vi "MyMethod2.vi"(0 "reference in":refnum<class "AnotherClass.lvclass">, 5 "error in (no error)":errorcluster) -> (14 "reference out":refnum<class "AnotherClass.lvclass">, 19 "error out":errorcluster)   [LabVIEW 2017, in "AnotherClass.lvclass"]
uses:
  AnotherClass.lvclass
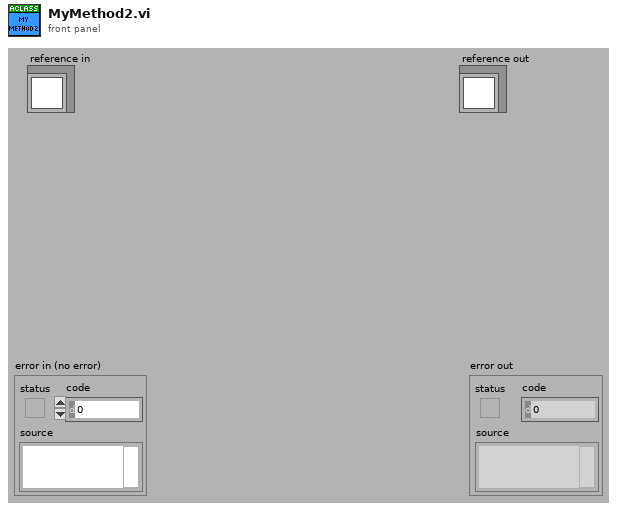
[diagram p1: front panel]
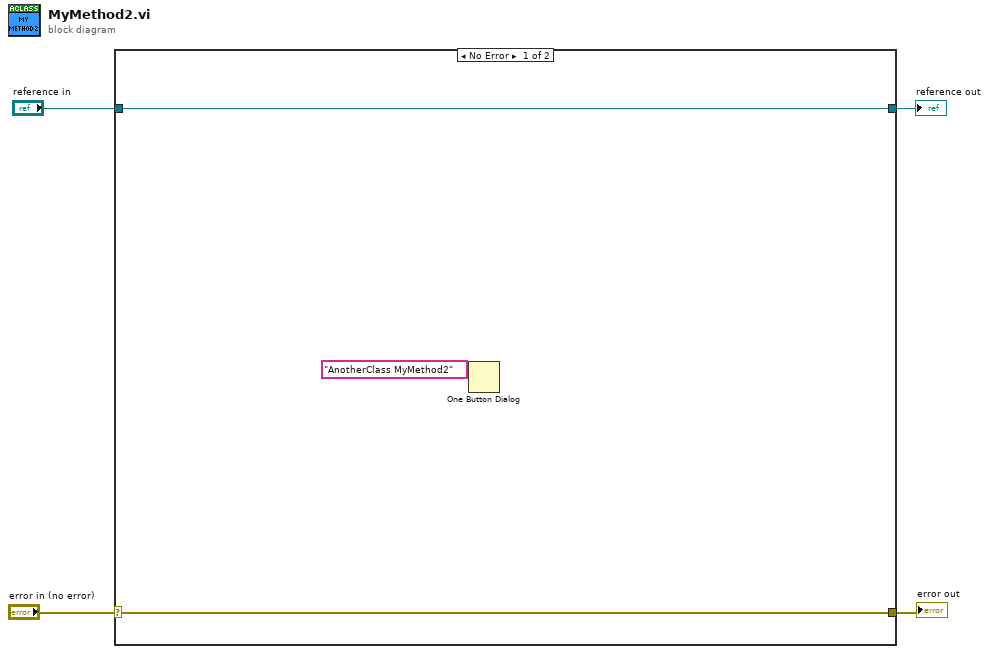
[diagram p0: block diagram]
diagram:
  n1 = case shown="No Error" "error in (no error)" {
    selector: "error in (no error)" -> [w6 w9]
    tunnel: [w6 w9] -> w3
    tunnel: [w7 w8] -> w1
    tunnel: "reference in" -> [w7 w8]
    frame No Error {
      n2 = One Button Dialog(message="AnotherClass MyMethod2") -> ()  [unwired: 2 out]
    }
    frame Error {
    }
  }
  "error out" <- w3
  "reference out" <- w1
